vi "Sort 2D Array__ogtk.vi"   [LabVIEW 2016]
doc: "This polymorphic VI sorts a 2D array of numerics or strings, regardless of the array size. You can specify whether to sort by column or row, which column or row to sort by, and whether to sort in ascending or descending order. You also can specify a secondary row or column to sort by."
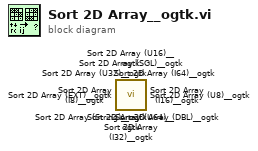
[diagram p0: block diagram]
diagram:
  n1 = call <userlib>:"Sort 2D Array (U64)__ogtk.vi"() -> ()  [unwired: 8 in, 4 out]
  n2 = call <userlib>:"Sort 2D Array (I64)__ogtk.vi"() -> ()  [unwired: 8 in, 4 out]
  n3 = call <userlib>:"Sort 2D Array (EXT)__ogtk.vi"() -> ()  [unwired: 8 in, 4 out]
  n4 = call <userlib>:"Sort 2D Array (U8)__ogtk.vi"() -> ()  [unwired: 8 in, 4 out]
  n5 = call <userlib>:"Sort 2D Array (U16)__ogtk.vi"() -> ()  [unwired: 8 in, 4 out]
  n6 = call <userlib>:"Sort 2D Array (U32)__ogtk.vi"() -> ()  [unwired: 8 in, 4 out]
  n7 = call <userlib>:"Sort 2D Array (I8)__ogtk.vi"() -> ()  [unwired: 8 in, 4 out]
  n8 = call <userlib>:"Sort 2D Array (I16)__ogtk.vi"() -> ()  [unwired: 8 in, 4 out]
  n9 = call <userlib>:"Sort 2D Array (I32)__ogtk.vi"() -> ()  [unwired: 8 in, 4 out]
  n10 = call <userlib>:"Sort 2D Array (DBL)__ogtk.vi"() -> ()  [unwired: 8 in, 4 out]
  n11 = call <userlib>:"Sort 2D Array (SGL)__ogtk.vi"() -> ()  [unwired: 8 in, 4 out]
  n12 = call <userlib>:"Sort 2D Array (String)__ogtk.vi"() -> ()  [unwired: 8 in, 4 out]
